vi "Send.vi"(8 "error in (no error)":errorcluster caption="错误输入（无错误）", 10 "数组":T1[](array[typedef]) {"Data" format="%x"; "ID" format="%x"}, 11 "ZLGCAN 输入":refnum<class "ZLGCAN.lvclass">) -> (0 "error out":errorcluster caption="错误输出", 3 "ZLGCAN 输出":refnum<class "ZLGCAN.lvclass">)   [LabVIEW 2020, in "ZLGCAN.lvclass"]
uses:
  ZLGCAN.lvclass
  CAN/CANData.ctl
  ZLGCAN.lvclass/ZLGCAN.ctl
  ControlCAN/VCI_CAN_OBJ.ctl
  CAN/CAN.lvclass
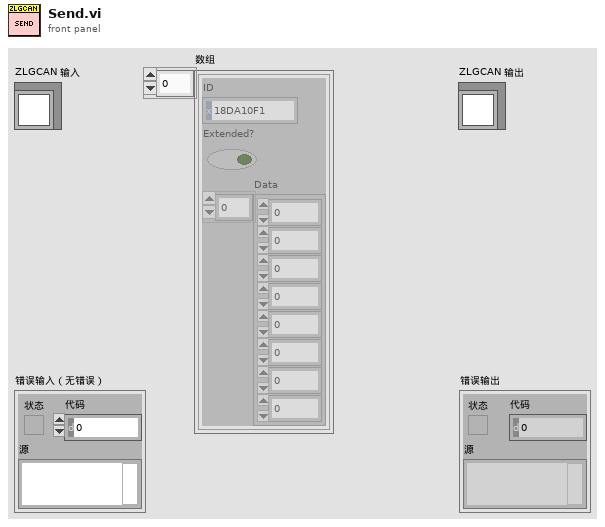
[diagram p1: front panel]
types:
  T1 = typedef "CAN.lvclass/CANData.ctl" = cluster{"ID":u32, "Extended?":bool, "Data":u8[]}
  T2 = typedef "ZLGCAN.lvclass/VCI_CAN_OBJ.ctl" = cluster{"ID":u32, "TimeStamp":u32, "TimeFlag":enum8{"invalid", "valid"}, "SendType":enum8{"Normal", "Once", "Test", "Once Test"}, "RemoteFlag":enum8{"Data", "Remote"}, "ExternFlag":enum8{"Standard", "Extern"}, "DataLen":u8, "Data0":u8, "Data1":u8, "Data2":u8, "Data3":u8, "Data4":u8, "Data5":u8, "Data6":u8, "Data7":u8, "Reserved0":u8, "Reserved1":u8, "Reserved2":u8}
  T3 = cluster{"Device Type":u32, "Device Index":u32, "CANInd":u32, "Baud(E_U)":u32}
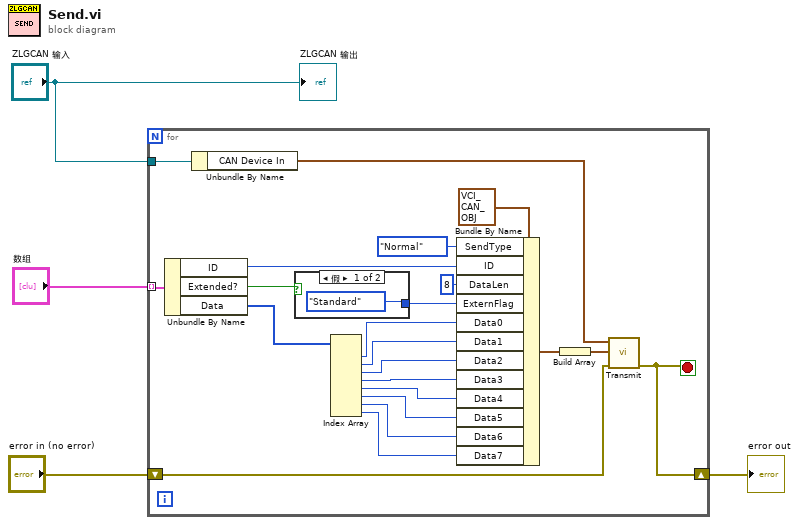
[diagram p0: block diagram]
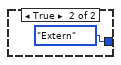
[diagram p2: hidden frame]
diagram:
  n1 = for {
    tunnel: "数组" -> [w12] mode=indexing
    shift-right: [w7] -> w2
    shift-left: "error in (no error)" -> [w8]
    tunnel: "ZLGCAN 输入" -> [w6]
    stop <- w7 stop-if-true
    n2 = Unbundle By Name(w12) -> ("ID"=w11:u32, "Extended?"=w10:bool, "Data"=w9:u8[])
    n3 = Unbundle By Name(w6) -> ("CAN Device In"=w5:T3)
    n4 = case shown="假" w10 {
      tunnel: [enum8{"Standard", "Extern"}."Standard" ("ExternFlag") enum8{"Standard", "Extern"}."Extern" ("ExternFlag")] -> w22
      frame False {
      }
      frame True {
      }
    }
    n5 = Index Array(array=w9) -> (element #1=w13:u8, element #2=w20:u8, element #3=w19:u8, element #4=w18:u8, element #5=w17:u8, element #6=w16:u8, element #7=w15:u8, element #8=w14:u8)  [unwired: 8 in]
    n6 = Bundle By Name(cluster=T2 {"ID"=0, "TimeStamp"=0, "TimeFlag"=enum."invalid", "SendType"=enum."Test", "RemoteFlag"=enum."Data", "ExternFlag"=enum."Standard", "DataLen"=0, "Data0"=0, "Data1"=0, "Data2"=0, "Data3"=0, "Data4"=0, "Data5"=0, "Data6"=0, "Data7"=0, "Reserved0"=0, "Reserved1"=0, "Reserved2"=0} ("pSend In"), "SendType"=enum8{"Normal", "Once", "Test", "Once Test"}."Normal", "ID"=w11, "DataLen"=u8 8, "ExternFlag"=w22, "Data0"=w13, "Data1"=w20, "Data2"=w19, "Data3"=w18, "Data4"=w17, "Data5"=w16, "Data6"=w15, "Data7"=w14) -> (w24:T2)
    n7 = Build Array(w24) -> (w23:T2[])
    n8 = call "Transmit.vi"("Error In(No Error)"=w8, "pSend In"=w23, "CAN Device In"=w5) -> ("Error Out"=w7:errorcluster)  [unwired: 5 in, 3 out]
  }
  "error out" <- w2
  "ZLGCAN 输出" <- "ZLGCAN 输入"
